vi "VNS Naderi Local Search Stand Alone.vi"() -> ()   [LabVIEW 2013]
uses:
  GA/Controls/Scheduler Type.ctl
  GA/Controls/Objective.ctl
  Classes/OSSP_Problem.lvclass
  Classes/OSSP_Problem.lvclass/OSSP_Problem.ctl
  Helper VIs/IRH Heuristic VIs/Initial Construction Heuristic.ctl
  Classes/Scheduler_Class/Operation to Machine Job Tuple.vi
  <vilib>/dlg_ctls.llb/Space Constant.vi
  Classes/Scheduler_Class/NonDelay Scheduler/Non Delay Scheduler Engine.vi
  Classes/Scheduler_Class/Prins FIFO Scheduler Methods and Controls/Prins FIFO Scheduler.vi
  Classes/Scheduler_Class/Prins FIFO Scheduler Methods and Controls/Methods/Calculate Final Completion Times of Jobs.vi
  GA/SubVIS/Calcualte General Tardiness.vi
  Helper VIs/IRH Heuristic VIs/LPTSequenceBulilder.vi
  Helper VIs/IRH Heuristic VIs/SPTSequenceBulilder.vi
  Helper VIs/IRH Heuristic VIs/EDDSequenceBulilder.vi
  Classes/Scheduler_Class/Giffler Thompson Active Schedule Engine.vi
  Classes/Scheduler_Class/Prins FIFO Scheduler Methods and Controls/Methods/Calculate Makespan (Prins FIFO Engine).vi
  Classes/Scheduler_Class/Prins FIFO Scheduler Methods and Controls/Methods/Calculate Tardiness (Prins FIFO Engine).vi
  Classes/Scheduler_Class/Modified GT Active Scheduler/GT Active Scheduler wSubset4Tardiness.vi
  GA/SubVIS/Remove Duplicates In Array.vi
  Classes/Scheduler_Class/Prins FIFO Scheduler Methods and Controls/Methods/Reorder Schedule(Prins FIFO) based on Start Times.vi
  Classes/Scheduler_Class/Prins FIFO Scheduler Methods and Controls/Methods/UpdateMachineGaps.vi
  Classes/Scheduler_Class/Prins FIFO Scheduler Methods and Controls/Methods/UpdateJobGaps.vi
  Classes/Scheduler_Class/Prins FIFO Scheduler Methods and Controls/Methods/Find Intersecting Gaps.vi
  Classes/Scheduler_Class/Modified GT Active Scheduler/GT Find Subset of Operations.vi
  Classes/Scheduler_Class/Modified GT Active Scheduler/Select Operation to Schedule Based on Rule.vi
  <vilib>/Analysis/1siggen.llb/Riffle Array (I32).vi
  Classes/Scheduler_Class/GT Algorithm Find M_ok and J_ok.vi
  Classes/Scheduler_Class/Prins FIFO Scheduler Methods and Controls/Methods/Transform to Plain Job and Machine Gaps Array.vi
  Classes/Scheduler_Class/Semiactive Scheduler/Semi Active Scheduler Engine.vi
  <vilib>/Analysis/NI_AALBase.lvlib
  Classes/Scheduler.lvclass
panel:
  in  "Objective":T1
  in  "Scheduler":T2
  in  "Reorder?":bool
  in  "Instance Number for Taillard":dbl
  in  "Problem Type":enum16{"Taillard", "Brucker", "Gueret Prins"}(ring)
  out "error out":errorcluster
  out "Tardiness(FIFO Engine)":u16
  out "VNS Result":u16[](array[numeric])
  out "Best Chromosome":u16[](array[numeric])
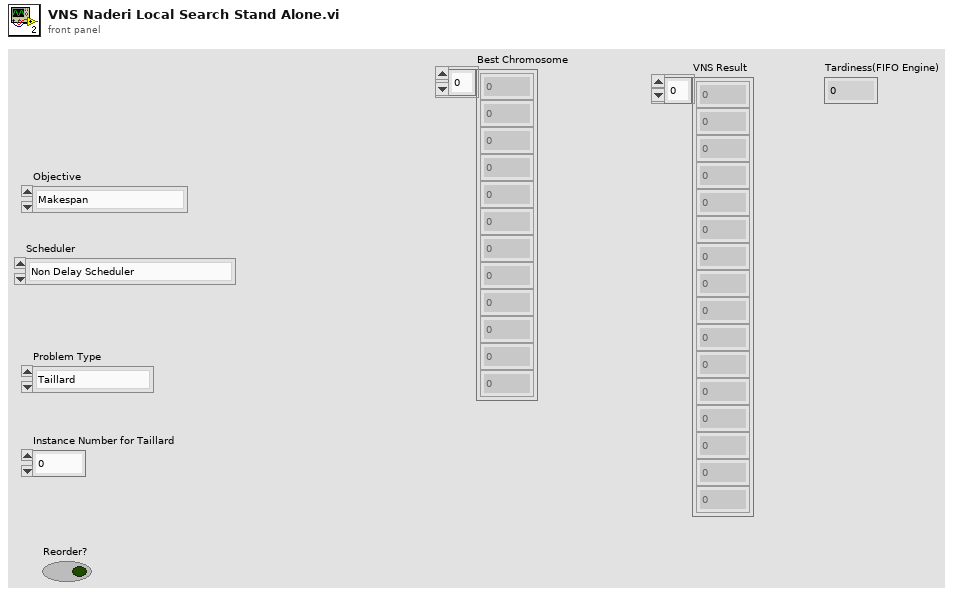
[diagram p1: front panel]
types:
  T1 = typedef "Objective.ctl" = enum16{"Makespan", "Total Tardiness"}
  T2 = typedef "Scheduler Type.ctl" = enum16{"Non Delay Scheduler", "GT Active Scheduler", "My Faulty Scheduler", "Prins FIFO Scheduler", "SemiActive Scheduler", "Modified GT Scheduler"}
  T3 = typedef "Initial Construction Heuristic.ctl" = enum16{"LPT", "SPT", "EDD"}
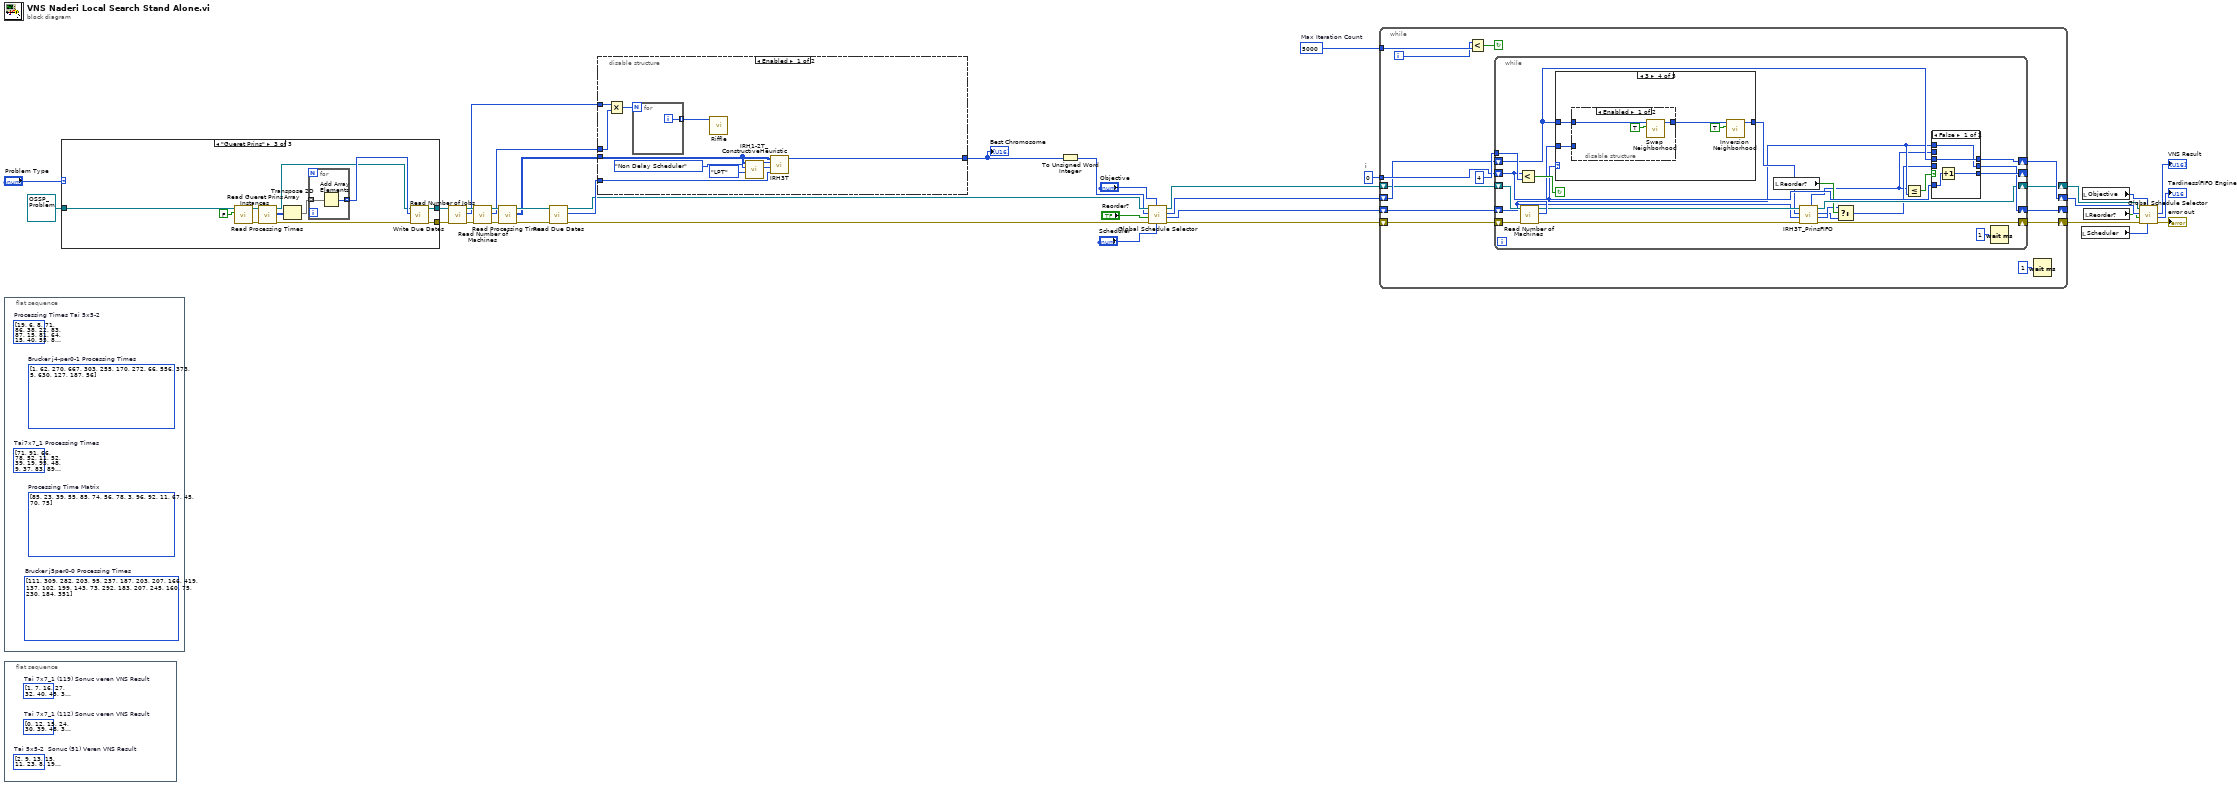
[diagram p0: block diagram]
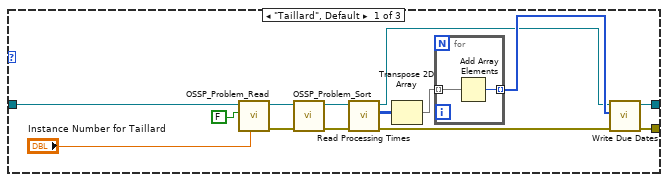
[diagram p2: hidden frame]
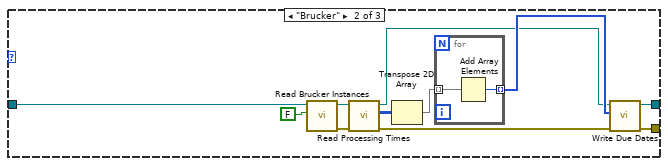
[diagram p3: hidden frame]
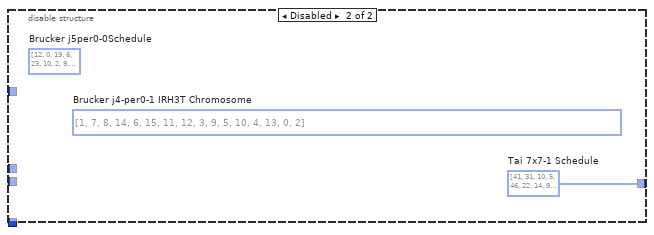
[diagram p4: hidden frame]
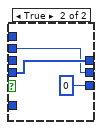
[diagram p5: hidden frame]
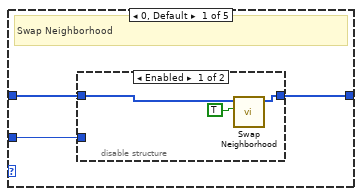
[diagram p6: hidden frame]
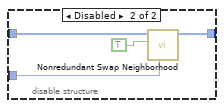
[diagram p7: hidden frame]
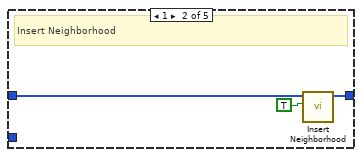
[diagram p8: hidden frame]
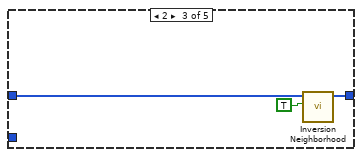
[diagram p9: hidden frame]
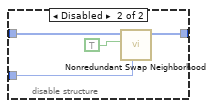
[diagram p10: hidden frame]
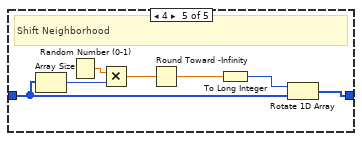
[diagram p11: hidden frame]
diagram:
  w35 = 0  # i
  w36 = 5000  # Max Iteration Count
  n1 = flat-sequence {
    frame #0 {
      (unwired) u16[][] [[1, 62, 270, 667], [303, 255, 170, 272], [66, 556, 373, 5], [630, 127, 187, 56]]  # Brucker j4-per0-1 Processing Times
      (unwired) u16[][] [[85, 23, 39, 55], [85, 74, 56, 78], [3, 96, 92, 11], [67, 45, 70, 75]]  # Processing Time Matrix
      (unwired) u16[][] [[19, 6, 8, 71, 86], [38, 22, 83, 87, 15], [81, 64, 15, 40, 55], [83, 90, 1, 21, 55], [32, 52, 35, 33, 42]]  # Processing Times Tai 5x5-2
      (unwired) u16[][] [[71, 91, 66, 78, 52, 11, 52], [39, 19, 95, 48, 9, 37, 83], [89, 13, 96, 19, 91, 30, 88], [54, 73, 18, 68, 28, 2, 45], [56, 46, 14, 63, 75, 98, 37], [92, 81, 48, 46, 60, 38, 52], [34, 27, 24, 94, 7, 33, 77]]  # Tai7x7_1 Processing Times
      (unwired) u16[][] [[111, 309, 282, 203, 95], [237, 187, 203, 207, 166], [419, 137, 102, 199, 143], [73, 292, 183, 207, 245], [160, 75, 230, 184, 351]]  # Brucker j5per0-0 Processing Times
    }
  }
  n2 = flat-sequence {
    frame #0 {
      (unwired) u16[] [2, 9, 13, 15, 11, 23, 8, 19, 0, 12, 21, 1, 10, 17, 14, 20, 4, 6, 18, 7, 16, 3, 24, 5, 22]  # Tai 5x5-2  Sonuc (51) Veren VNS Result
      (unwired) u16[] [0, 12, 15, 24, 30, 39, 48, 3, 27, 7, 47, 16, 32, 36, 1, 38, 40, 45, 25, 6, 29, 35, 10, 43, 28, 19, 37, 41, 4, 23, 14, 33, 9, 22, 13, 44, 11, 5, 31, 20, 21, 17, 34, 8, 18, 46, 2, 26, 42]  # Tai 7x7_1 (112) Sonuc veren VNS Result
      (unwired) u16[] [1, 7, 16, 27, 32, 40, 45, 36, 3, 47, 29, 39, 15, 30, 12, 48, 0, 24, 6, 25, 38, 35, 10, 28, 37, 19, 43, 41, 4, 23, 14, 33, 9, 13, 22, 44, 11, 5, 31, 20, 21, 17, 34, 8, 18, 46, 2, 26, 42]  # Tai 7x7_1 (119) Sonuc veren VNS Result
    }
  }
  n3 = case shown="\"Gueret Prins\"" "Problem Type" {
    tunnel: refnum<class "OSSP_Problem.lvclass"> refnum ("OSSP_Problem.lvclass") -> [w50 w63 w76]
    tunnel: [w43 w58 w71] -> w32
    tunnel: [w42 w59 w72] -> w31
    frame "Taillard", Default {
      n4 = call "OSSP_Problem_Read.vi"("Instance Number"="Instance Number for Taillard", "Auto Mode"=FALSE, "OSSP_Problem.lvclass In"=w50) -> ("error out"=w47:errorcluster, "OSSP_Problem.lvclass Out"=w48:refnum<class "OSSP_Problem.lvclass">)  [unwired: 7 in]
      n5 = call "OSSP_Problem_Sort.vi"("error in (no error)"=w47, "OSSP_Problem.lvclass In"=w48) -> ("error out"=w45:errorcluster, "OSSP_Problem.lvclass Out"=w44:refnum<class "OSSP_Problem.lvclass">)  [unwired: 8 in]
      n6 = call "Read Processing Times.vi"("error in (no error)"=w45, "OSSP_Problem in"=w44) -> ("error out"=w37:errorcluster, "Processing Times"=w40:u16[][], "OSSP_Problem out"=w38:refnum<class "OSSP_Problem.lvclass">)  [unwired: 7 in]
      n7 = Transpose 2D Array(2D array=w40) -> (transposed array=w41:u16[][])
      n8 = for {
        tunnel: w41 -> [w52] mode=indexing
        tunnel: [w51] -> w39 mode=indexing
        n9 = Add Array Elements(numeric array=w52) -> (sum=w51:u16)
      }
      n10 = call "Write Due Dates.vi"("error in (no error)"=w37, "Due Dates"=w39, "OSSP_Problem in"=w38) -> ("error out"=w42:errorcluster, "OSSP_Problem out"=w43:refnum<class "OSSP_Problem.lvclass">)  [unwired: 7 in]
    }
    frame "Brucker" {
      n11 = call "Read Brucker Instances.vi"("Auto Mode"=FALSE, "OSSP_Problem in"=w63) -> ("error out"=w60:errorcluster, "OSSP_Problem out"=w61:refnum<class "OSSP_Problem.lvclass">)  [unwired: 8 in]
      n12 = call "Read Processing Times.vi"("error in (no error)"=w60, "OSSP_Problem in"=w61) -> ("error out"=w53:errorcluster, "Processing Times"=w56:u16[][], "OSSP_Problem out"=w54:refnum<class "OSSP_Problem.lvclass">)  [unwired: 7 in]
      n13 = Transpose 2D Array(2D array=w56) -> (transposed array=w57:u16[][])
      n14 = for {
        tunnel: w57 -> [w65] mode=indexing
        tunnel: [w64] -> w55 mode=indexing
        n15 = Add Array Elements(numeric array=w65) -> (sum=w64:u16)
      }
      n16 = call "Write Due Dates.vi"("error in (no error)"=w53, "Due Dates"=w55, "OSSP_Problem in"=w54) -> ("error out"=w59:errorcluster, "OSSP_Problem out"=w58:refnum<class "OSSP_Problem.lvclass">)  [unwired: 7 in]
    }
    frame "Gueret Prins" {
      n17 = call "Read Gueret Prins Instances.vi"("Auto Mode"=FALSE, "OSSP_Problem in"=w76) -> ("error out"=w73:errorcluster, "OSSP_Problem out"=w74:refnum<class "OSSP_Problem.lvclass">)  [unwired: 8 in]
      n18 = call "Read Processing Times.vi"("error in (no error)"=w73, "OSSP_Problem in"=w74) -> ("error out"=w66:errorcluster, "Processing Times"=w69:u16[][], "OSSP_Problem out"=w67:refnum<class "OSSP_Problem.lvclass">)  [unwired: 7 in]
      n19 = Transpose 2D Array(2D array=w69) -> (transposed array=w70:u16[][])
      n20 = for {
        tunnel: w70 -> [w78] mode=indexing
        tunnel: [w77] -> w68 mode=indexing
        n21 = Add Array Elements(numeric array=w78) -> (sum=w77:u16)
      }
      n22 = call "Write Due Dates.vi"("error in (no error)"=w66, "Due Dates"=w68, "OSSP_Problem in"=w67) -> ("error out"=w72:errorcluster, "OSSP_Problem out"=w71:refnum<class "OSSP_Problem.lvclass">)  [unwired: 7 in]
    }
  }
  n23 = call "Read Number of Jobs.vi"("error in (no error)"=w31, "OSSP_Problem in"=w32) -> ("error out"=w29:errorcluster, "Number of Jobs"=w24:i32, "OSSP_Problem out"=w30:refnum<class "OSSP_Problem.lvclass">)  [unwired: 7 in]
  n24 = call "Read Number of Machines.vi"("error in (no error)"=w29, "OSSP_Problem in"=w30) -> ("error out"=w27:errorcluster, "Number of Machines"=w23:i32, "OSSP_Problem out"=w28:refnum<class "OSSP_Problem.lvclass">)  [unwired: 7 in]
  n25 = call "Read Processing Times.vi"("error in (no error)"=w27, "OSSP_Problem in"=w28) -> ("error out"=w25:errorcluster, "Processing Times"=w21:u16[][], "OSSP_Problem out"=w26:refnum<class "OSSP_Problem.lvclass">)  [unwired: 7 in]
  n26 = call "Read Due Dates.vi"("error in (no error)"=w25, "OSSP_Problem in"=w26) -> ("error out"=w15:errorcluster, "Due Dates"=w20:u16[], "OSSP_Problem out"=w19:refnum<class "OSSP_Problem.lvclass">)  [unwired: 7 in]
  n27 = disable-structure shown="Enabled" {
    disable-tunnel: [w79 w91] -> w34
    disable-tunnel: w24 -> [w88 _]
    disable-tunnel: w23 -> [w87 _]
    disable-tunnel: w21 -> [w82 _]
    disable-tunnel: w20 -> [w80 _]
    frame Enabled {
      n28 = Multiply(x=w88, y=w87) -> (x*y=w86:i32)
      n29 = for {
        N: w86 -> [_]
        tunnel: [w90] -> w89 mode=indexing
        i -> [w90]
      }
      n30 = call-poly <vilib>:"Riffle.vi"("X"=w89) -> ()  [unwired: 8 in, 3 out]
      n31 = call "IRH1-2T_ConstructiveHeuristic.vi"("Initial Construction Heursitic"=Initial_Construction_Heuristic."LPT", "Scheduler"=Scheduler_Type."Non Delay Scheduler", "Proocessing Times MxJ"=w82) -> ("Total Tardiness"=w81:u16, "IRH2T Schedule Out"=w83:u16[])  [unwired: 6 in, 1 out]
      n32 = call "IRH3T.vi"("Due Dates"=w80, "Initial Tardiness"=w81, "Schedule 2B Improved"=w83, "Proocessing Times  (Machines x Jobs)"=w82) -> ("IRH3T (Reordered) Schedule Out"=w79:u16[])  [unwired: 5 in, 2 out]
    }
    frame Disabled {
      w91 = i32[] [41, 31, 10, 5, 46, 22, 14, 9, 30, 39, 48, 21, 15, 3, 12, 34, 44, 32, 35, 27, 0, 38, 17, 36, 19, 8, 45, 37, 11, 29, 1, 28, 18, 16, 40, 23, 24, 13, 4, 43, 33, 7, 6, 25, 47, 2, 20, 42, 26]  # Tai 7x7-1 Schedule
      (unwired) i32[] [12, 0, 19, 6, 23, 10, 2, 9, 16, 8, 24, 11, 15, 7, 3, 20, 14, 18, 1, 5, 22, 13, 17, 21, 4]  # Brucker j5per0-0Schedule
      (unwired) i32[] [1, 7, 8, 14, 6, 15, 11, 12, 3, 9, 5, 10, 4, 13, 0, 2]  # Brucker j4-per0-1 IRH3T Chromosome
    }
  }
  "Best Chromosome" <- w34
  n33 = To Unsigned Word Integer(number=w34) -> (unsigned 16bit integer=w18:u16[])
  n34 = call "Global Schedule Selector.vi"("Scheduler"="Scheduler", "Objective"="Objective", "error in (no error)"=w15, "Reorder?"="Reorder?", "Schedule in"=w18, "OSSP_Problem in"=w19) -> ("error out"=w14:errorcluster, "Total Tardiness or Makespan (U16)"=w13:u16, "Schedule out"=w17:u16[], "OSSP_Problem out"=w16:refnum<class "OSSP_Problem.lvclass">)  [unwired: 2 in]
  n35 = while {
    tunnel: w36 -> [w105]
    tunnel: w35 -> [w102]
    shift-right: [w100] -> w6
    shift-left: w17 -> [w99]
    shift-right: [w97] -> _
    shift-left: w13 -> [w98]
    shift-right: [w94] -> w9
    shift-left: w16 -> [w96]
    shift-right: [w93] -> w7
    shift-left: w14 -> [w95]
    i -> [w101]
    stop <- w104 continue-if-true
    n36 = Less?(x=w101, y=w105) -> (x < y?=w104:bool)
    n37 = while {
      tunnel: 4 -> [w126]
      shift-right: [w125] -> _
      shift-left: w102 -> [w122]
      shift-right: [w124] -> w100
      shift-left: w99 -> [w123]
      shift-right: [w121] -> w97
      shift-left: w98 -> [w113]
      shift-right: [w115] -> w94
      shift-left: w96 -> [w117]
      shift-right: [w111] -> w93
      shift-left: w95 -> [w118]
      stop <- w128 continue-if-true
      n38 = Less?(x=w122, y=w126) -> (x < y?=w128:bool)
      n39 = call "Read Number of Machines.vi"("error in (no error)"=w118, "OSSP_Problem in"=w117) -> ("error out"=w112:errorcluster, "Number of Machines"=w120:i32, "OSSP_Problem out"=w116:refnum<class "OSSP_Problem.lvclass">)  [unwired: 7 in]
      n40 = case shown="3" w122 {
        tunnel: w123 -> [w138 w148 w151 w156 w166]
        tunnel: [w137 w147 w150 w154 w165] -> w114
        tunnel: w120 -> [w136 _ _ w152 _]
        frame 0, Default {
          # "Swap Neighborhood"
          n41 = disable-structure shown="Enabled" {
            disable-tunnel: w138 -> [w141 w145]
            disable-tunnel: [w140 w144] -> w137
            disable-tunnel: w136 -> [_ w142]
            frame Enabled {
              n42 = call "Swap Neighborhood.vi"("Generate Random Indices?"=TRUE, "Schedule In"=w141) -> ("Schedule Out"=w140:u16[])  [unwired: 9 in]
            }
            frame Disabled {
              n43 = call "Nonredundant Swap Neighborhood.vi"("Number of Machines"=w142, "Generate Random indices?"=TRUE, "Schedule in"=w145) -> ("Schedule out"=w144:u16[])  [unwired: 8 in]
            }
          }
        }
        frame 1 {
          # "Insert Neighborhood"
          n44 = call "Insert Neighborhood.vi"("Generate Random Indices?"=TRUE, "C'"=w148) -> ("Chromosome Out"=w147:u16[])  [unwired: 9 in]
        }
        frame 2 {
          n45 = call "Inversion Neighborhood.vi"("Generate Random Indices?"=TRUE, "Schedule in"=w151) -> ("Schedule out"=w150:u16[])  [unwired: 9 in]
        }
        frame 3 {
          n46 = disable-structure shown="Enabled" {
            disable-tunnel: w156 -> [w159 w163]
            disable-tunnel: [w158 w162] -> w155
            disable-tunnel: w152 -> [_ w160]
            frame Enabled {
              n47 = call "Swap Neighborhood.vi"("Generate Random Indices?"=TRUE, "Schedule In"=w159) -> ("Schedule Out"=w158:u16[])  [unwired: 9 in]
            }
            frame Disabled {
              n48 = call "Nonredundant Swap Neighborhood.vi"("Number of Machines"=w160, "Generate Random indices?"=TRUE, "Schedule in"=w163) -> ("Schedule out"=w162:u16[])  [unwired: 8 in]
            }
          }
          n49 = call "Inversion Neighborhood.vi"("Generate Random Indices?"=TRUE, "Schedule in"=w155) -> ("Schedule out"=w154:u16[])  [unwired: 9 in]
        }
        frame 4 {
          # "Shift Neighborhood"
          n50 = Array Size(array=w166) -> (size(s)=w169:i32)
          n51 = Random Number (0-1)() -> (number: 0 to 1=w170:dbl)
          n52 = Multiply(x=w170, y=w169) -> (x*y=w168:dbl)
          n53 = Round Toward -Infinity(1:w168) -> (0:w167:dbl)
          n54 = To Long Integer(number=w167) -> (32bit integer=w164:i32)
          n55 = Rotate 1D Array(1:w166, 2:w164) -> (0:w165:u16[])
        }
      }
      n56 = local read "Reorder?"() -> (w110:bool)
      n57 = call "IRH3T_PrinsFIFO.vi"("error in (no error)"=w112, "Initial Tardiness"=w113, "Schedule 2B Improved"=w114, "OSSP_Problem.lvclass"=w116) -> ("error out"=w111:errorcluster, "IRH3T (Reordered) Schedule Out"=w109:u16[], "IRH3T Schedule Out"=w108:u16[], "OSSP_Problem out"=w115:refnum<class "OSSP_Problem.lvclass">, "Total Tardiness"=w106:u16)  [unwired: 3 in]
      n58 = Select(t=w109, s=w110, f=w108) -> (s? t:f=w107:u16[])
      n59 = Less Or Equal?(x=w106, y=w113) -> (x <= y?=w127:bool)
      n60 = case shown="False" w127 {
        tunnel: w122 -> [w131 _]
        tunnel: w107 -> [_ w134]
        tunnel: [w132 0] -> w125
        tunnel: [w130 w134] -> w124
        tunnel: w123 -> [w130 _]
        tunnel: w106 -> [_ w133]
        tunnel: [w129 w133] -> w121
        tunnel: w113 -> [w129 _]
        frame False {
          n61 = Increment(x=w131) -> (x+1=w132:i32)
        }
        frame True {
        }
      }
      n62 = Wait (ms)(milliseconds to wait=u32 1) -> ()  [unwired: 1 out]
    }
    n63 = Wait (ms)(milliseconds to wait=u32 1) -> ()  [unwired: 1 out]
  }
  n64 = local read "Scheduler"() -> (w1:T2)
  n65 = local read "Objective"() -> (w3:T1)
  n66 = local read "Reorder?"() -> (w2:bool)
  n67 = call "Global Schedule Selector.vi"("Scheduler"=w1, "Objective"=w3, "error in (no error)"=w7, "Reorder?"=w2, "Schedule in"=w6, "OSSP_Problem in"=w9) -> ("error out"=→"error out":errorcluster, "Total Tardiness or Makespan (U16)"=→"Tardiness(FIFO Engine)":u16, "Schedule out"=→"VNS Result":u16[])  [unwired: 2 in, 1 out]
